vi "T1 Parametric Testing.vi"(8 "error in (no error)":errorcluster, 9 "Operator":string, 10 "table name":string="Test_Results", 11 "connection reference":T1) -> (0 "error out":errorcluster, 3 "connection reference out":T1)   [LabVIEW 2023]
doc: "The T1 Parametric testing application performs parametric testing of T1 signals. The T1 signal is a 1.544 Mb/s pulsed digital signal formed by multiplexing 24 voice channels. Each channel is sampled at 8000 samples/sec. Each sample is then converted to 8 bits using Pulse Coded Multiplexing. The 24 channels are then time-division multiplexed. Each frame, which corresponds to one sampling period, contains 192 bits ( 8 times 24) plus one bit for frame synchronization. Since frames occur at 8000 times per second, the bit rate is 1.544 Mb/s\n\nThis application performs the following parametric tests on T1 signals:\n\n1. Mask Test: Compares T1 signals with standard masks. The type of masks that are supported are ITU G.703 mask, EIA/TIA 547 and ANSI T1.102. The graph shows the mask in grey, the actual signal in green and failures as red squares. A boolean indicates whether the signal passed or failed the mask test and the indicator Number of Hits shows the number of times the signal did not pass the mask test.\n\n2. Measure T1 signal amplitude : Measures the amplitude of the T1 signal. The peak amplitude is displayed in the indicator Measured Amplitude.\n\n3. Measure T1 signal frequency : Measures the frequency of the T1 signal. The signal frequency in MHz is displayed in the indicator Measured Frequency."
uses:
  <vilib>/addons/database/Connection.llb/Conn ObjectReference.ctl
  <vilib>/addons/database/Auxilliary.llb/DB Tools Column Info.ctl
  <vilib>/addons/database/Auxilliary.llb/DB Tools DataTypes.ctl
  <vilib>/addons/database/NI_Database_API.lvlib
panel:
  out "Fail":bool
  in  "Log to Database":bool
  in  "Start Testing":bool
  out "Standard":string
  out "Date/Time":string
  out "UUT Serial #":string
  out "Failures":i32(slide) scale=0.0..10.0
  out "Tests":i32(slide) scale=0.0..10.0
  in  "quit":bool
  out "Amplitude (Vrms)":dbl(knob) scale=0.0..3.0
  in  "Polarity":u16(ring) items=["Positive", "Negative"]
  out "Frequency (MHz)":dbl format="%.4f"
  out "Time Domain Signal":waveform(dbl)(graph)
  out "Amplitude Spectrum":T2(graph)
  out "Signal Mask Test":waveform(dbl)[](graph)
  # "Telecommunications Parametric Testing"
  # "Instructions: Click Start Testing, then Log to Database, then Quit."
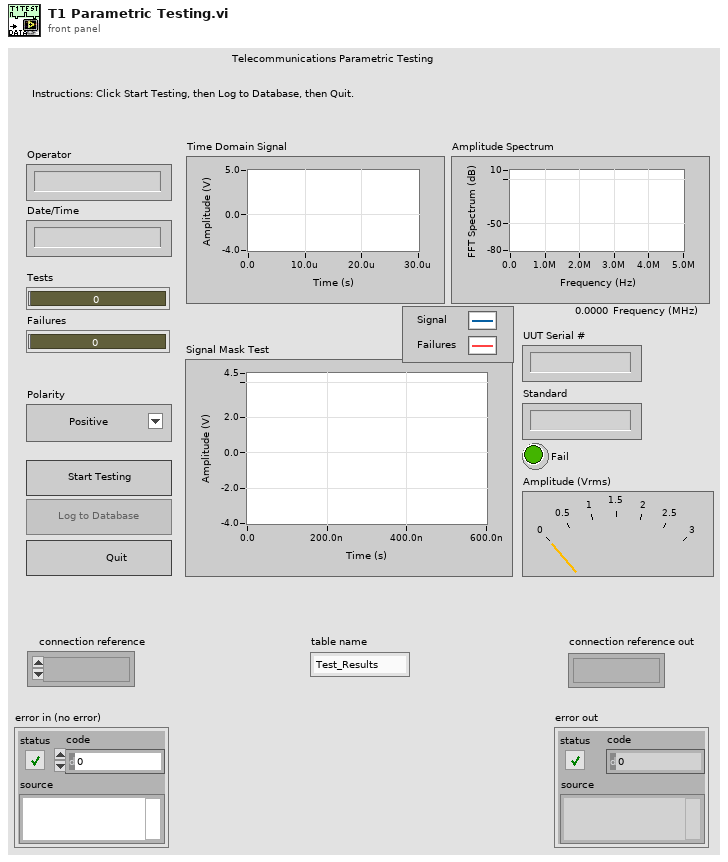
[diagram p1: front panel]
types:
  T1 = typedef "NI_Database_API.lvlib/Conn ObjectReference.ctl" = refnum<k1>
  T2 = cluster{"f0":dbl, "df":dbl, "dB Spectrum (Hann)":dbl[]}
  T3 = enum8{"Enabled", "Disabled", "Disabled and Grayed Out"}
  T4 = typedef "NI_Database_API.lvlib/DB Tools Column Info.ctl" = cluster{"column name":string, "data type":T5, "size":i32, "allow null?":bool}
  T5 = typedef "NI_Database_API.lvlib/DB Tools DataTypes.ctl" = enum16{"String", "Long (I32)", "Single (SGL)", "Double (DBL)", "Date/Time", "Binary"}
  T6 = cluster{"Time Domain Signal":waveform(dbl), "Signal Mask Test":waveform(dbl)[], "Amplitude (Vrms)":dbl, "Frequency (MHz)":dbl, "Date/Time":string, "Passed?":bool}
  T7 = cluster{"Operator":string, "Date/Time":string, "Date/Time":string, "Date/Time":string, "Frequency (MHz)":dbl, "Date/Time":string, "Date/Time":string}
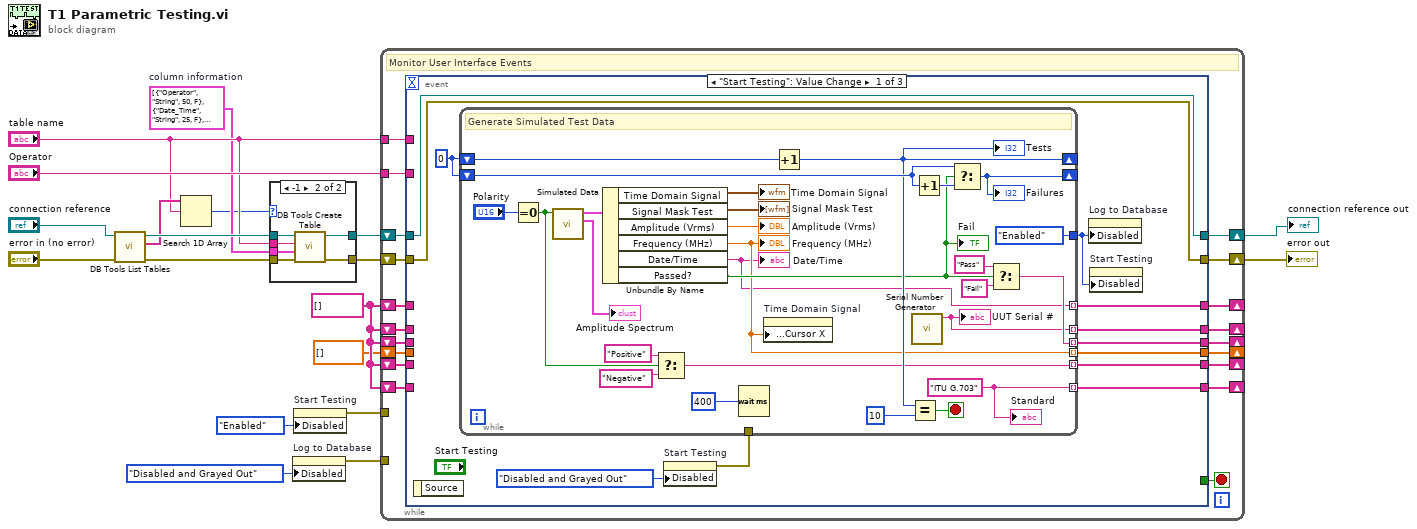
[diagram p0: block diagram]
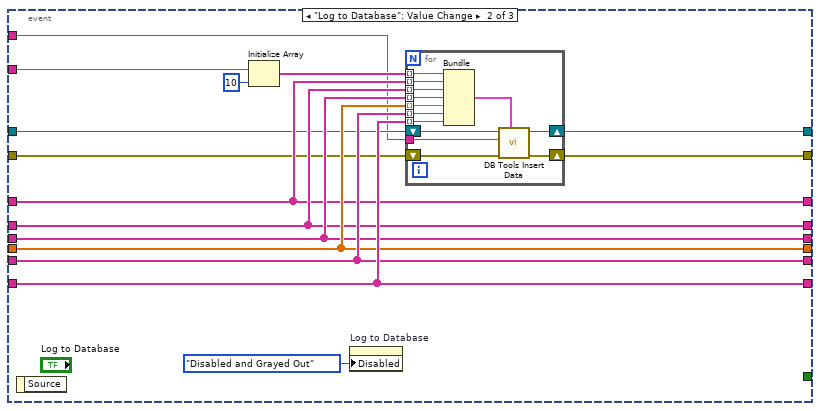
[diagram p3: hidden frame]
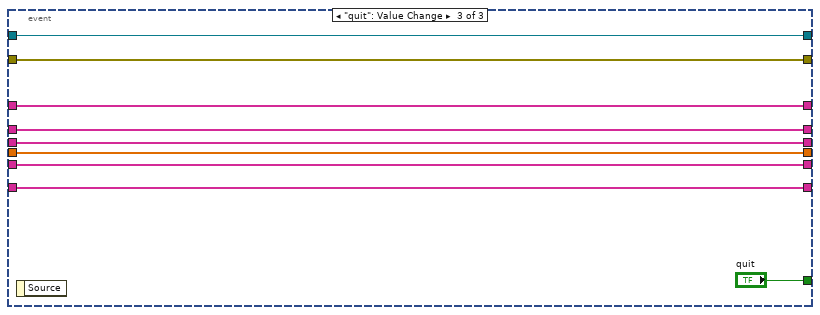
[diagram p4: hidden frame]
diagram:
  w6 = T4[] [{"column name"="Operator", "data type"=enum."String", "size"=50, "allow null?"=FALSE}, {"column name"="Date_Time", "data type"=enum."String", "size"=25, "allow null?"=FALSE}, {"column name"="UUT_Serial_Num", "data type"=enum."String", "size"=13, "allow null?"=FALSE}, {"column name"="Pass_Fail", "data type"=enum."String", "size"=4, "allow null?"=FALSE}, {"column name"="Frequency", "data type"=enum."Double (DBL)", "size"=0, "allow null?"=FALSE}, {"column name"="Polarity", "data type"=enum."String", "size"=8, "allow null?"=FALSE}, {"column name"="Standard", "data type"=enum."String", "size"=9, "allow null?"=FALSE}]  # column information
  w10 = string[] []
  n1 = call <vilib>:"DB Tools List Tables.vi"("error in (no error)"="error in (no error)", "connection reference"="connection reference") -> ("error out"=w15:errorcluster, "tables"=w12:string[], "connection reference out"=w13:T1)  [unwired: 3 in]
  n2 = Search 1D Array(1D array=w12, element="table name") -> (index of element=w5:i32)  [unwired: 1 in]
  n3 = case shown="-1" w5 {
    tunnel: w15 -> [w20 w27]
    tunnel: w13 -> [w21 w26]
    tunnel: "table name" -> [_ w25]
    tunnel: [w20 w24] -> w8
    tunnel: [w21 w23] -> w7
    tunnel: w6 -> [_ w22]
    frame Default {
    }
    frame -1 {
      n4 = call <vilib>:"DB Tools Create Table.vi"("error in (no error)"=w27, "column information"=w22, "table"=w25, "connection reference"=w26) -> ("error out"=w24:errorcluster, "connection reference out"=w23:T1)  [unwired: 4 in]
    }
  }
  n5 = property on="Log to Database" class="Bool"("Disabled"=T3."Disabled and Grayed Out") -> (error out=w3:errorcluster)  [unwired: 2 in, 1 out]
  n6 = property on="Start Testing" class="Bool"("Disabled"=T3."Enabled") -> (error out=w4:errorcluster)  [unwired: 2 in, 1 out]
  n7 = while {
    shift-right: [w45] -> _
    shift-left: w10 -> [w39]
    shift-right: [w44] -> _
    shift-left: w10 -> [w38]
    shift-right: [w43] -> _
    shift-left: w10 -> [w37]
    shift-right: [w42] -> _
    shift-left: dbl[] [] -> [w36]
    shift-right: [w41] -> _
    shift-left: w10 -> [w35]
    shift-right: [w40] -> _
    shift-left: w10 -> [w34]
    shift-right: [w31] -> w18
    shift-left: w7 -> [w30]
    shift-right: [w32] -> w19
    shift-left: w8 -> [w33]
    tunnel: "Operator" -> [w29]
    tunnel: "table name" -> [w28]
    tunnel: w4 -> [_]
    tunnel: w3 -> [_]
    stop <- w46 stop-if-true
    # "Monitor User Interface Events"
    n8 = event shown="[0] \"Start Testing\": Value Change" {
      selector: _ -> [_ _ _]
      dyn-events: _ -> [_ _ _]
      timeout: _ -> [_ _ _]
      tunnel: [_ _ "quit"] -> w46
      tunnel: [w57 w93 w122] -> w45
      tunnel: [w56 w94 w121] -> w44
      tunnel: [w55 w95 w120] -> w43
      tunnel: [w54 w96 w119] -> w42
      tunnel: [w53 w97 w118] -> w41
      tunnel: [w52 w98 w117] -> w40
      tunnel: w39 -> [_ w93 w122]
      tunnel: w38 -> [_ w94 w121]
      tunnel: w37 -> [_ w95 w120]
      tunnel: w36 -> [_ w96 w119]
      tunnel: w35 -> [_ w97 w118]
      tunnel: w34 -> [_ w98 w117]
      tunnel: w33 -> [w47 w92 w114]
      tunnel: [w47 w91 w114] -> w32
      tunnel: [w48 w90 w115] -> w31
      tunnel: w30 -> [w48 w89 w115]
      tunnel: w29 -> [_ w87 _]
      tunnel: w28 -> [_ w86 _]
      event "Start Testing": Value Change {
        w50 = 0
        n9 = event-data() -> ()  [unwired: 1 in, 1 out]
        n10 = property on="Start Testing" class="Bool"("Disabled"=T3."Disabled and Grayed Out") -> (error out=w49:errorcluster)  [unwired: 2 in, 1 out]
        n11 = while {
          tunnel: [w61] -> w54 mode=indexing
          tunnel: [w60] -> w57 mode=indexing
          tunnel: [w84] -> w52 mode=indexing
          tunnel: [w76] -> w53 mode=indexing
          tunnel: [w71] -> w55 mode=indexing
          tunnel: [w59] -> w56 mode=indexing
          shift-left: w50 -> [w81]
          shift-right: [w80] -> _
          shift-left: w50 -> [w82]
          shift-right: [w68] -> _
          tunnel: [T3."Enabled" ("Disabled")] -> w51
          tunnel: w49 -> [_]
          stop <- w85 stop-if-true
          w84 = "ITU G.703" ("Standard")
          # "Generate Simulated Test Data"
          n12 = Equal To 0?(x="Polarity") -> (x = 0?=w67:bool)
          n13 = call "Simulated Data.vi"("Polarity"=w67) -> ("Amplitude Spectrum"=→"Amplitude Spectrum":T2, "Cluster"=w78:T6)  [unwired: 9 in]
          n14 = Unbundle By Name(w78) -> ("Time Domain Signal"=→"Time Domain Signal":waveform(dbl), "Signal Mask Test"=→"Signal Mask Test":waveform(dbl)[], "Amplitude (Vrms)"=→"Amplitude (Vrms)":dbl, "Frequency (MHz)"=w61:dbl, "Date/Time"=w60:string, "Passed?"=w72:bool)
          "Frequency (MHz)" <- w61
          "Fail" <- w72
          "Date/Time" <- w60
          n15 = Select(t="Positive", s=w67, f="Negative") -> (s? t:f=w76:string)
          n16 = Wait (ms)(milliseconds to wait=u32 400) -> ()  [unwired: 1 out]
          n17 = property on="Time Domain Signal" class="WFGraph (strict)"("Cursor.Cursor Position:Cursor X"=w61) -> ()  [unwired: 2 in, 2 out]
          n18 = Increment(x=w81) -> (x+1=w80:i32)
          "Tests" <- w80
          n19 = Equal?(x=w80, y=10) -> (x = y?=w85:bool)
          n20 = call "Serial Number Generator.vi"() -> ("UUT Serial #"=w59:string)  [unwired: 11 in]
          "UUT Serial #" <- w59
          n21 = Increment(x=w82) -> (x+1=w83:i32)
          n22 = Select(t=w82, s=w72, f=w83) -> (s? t:f=w68:i32)
          "Failures" <- w68
          n23 = Select(t="Pass", s=w72, f="Fail") -> (s? t:f=w71:string)
          "Standard" <- w84
        }
        n24 = property on="Log to Database" class="Bool"("Disabled"=w51) -> ()  [unwired: 2 in, 2 out]
        n25 = property on="Start Testing" class="Bool"("Disabled"=w51) -> ()  [unwired: 2 in, 2 out]
      }
      event "Log to Database": Value Change {
        n26 = event-data() -> ()  [unwired: 1 in, 1 out]
        n27 = Initialize Array(w87, 10 ("Dimension Size")) -> (w100:string[])
        n28 = property on="Log to Database" class="Bool"("Disabled"=T3."Disabled and Grayed Out") -> ()  [unwired: 2 in, 2 out]
        n29 = for {
          tunnel: w100 -> [w110] mode=indexing
          tunnel: w93 -> [w109] mode=indexing
          tunnel: w94 -> [w108] mode=indexing
          tunnel: w95 -> [w107] mode=indexing
          tunnel: w96 -> [w106] mode=indexing
          tunnel: w97 -> [w105] mode=indexing
          tunnel: w98 -> [w104] mode=indexing
          tunnel: w86 -> [w101]
          shift-right: [w111] -> w91
          shift-left: w92 -> [w102]
          shift-right: [w112] -> w90
          shift-left: w89 -> [w103]
          n30 = Bundle("Operator"=w110, "Date/Time"=w109, "Date/Time"=w108, "Date/Time"=w107, "Frequency (MHz)"=w106, "Date/Time"=w105, "Date/Time"=w104) -> (w113:T7)  [unwired: 1 in]
          n31 = call <vilib>:"DB Tools Insert Data.vi"("data"=w113, "error in (no error)"=w102, "table"=w101, "connection reference"=w103) -> ("error out"=w111:errorcluster, "connection reference out"=w112:T1)  [unwired: 6 in]
        }
      }
      event "quit": Value Change {
        n32 = event-data() -> ()  [unwired: 1 in, 1 out]
      }
    }
  }
  "connection reference out" <- w18
  "error out" <- w19
